vi "closeMethodViReference.vi"(8 "error in (no error)":errorcluster, 11 "TestCase in":refnum<class "TestCase.lvclass">) -> (0 "error out":errorcluster, 3 "TestCase in":refnum<class "TestCase.lvclass">)   [LabVIEW 2011, in "TestCase.lvclass"]
uses:
  TestCase.lvclass
  TestCase.lvclass/TestCase.ctl
panel:
  # "JKI VI Tester for LabVIEW\nhttp://jkisoft.com/vi-tester\nCopyright (C) 2007-2009, JKI <info@jkisoft.com>\nALL RIGHTS RESERVED"
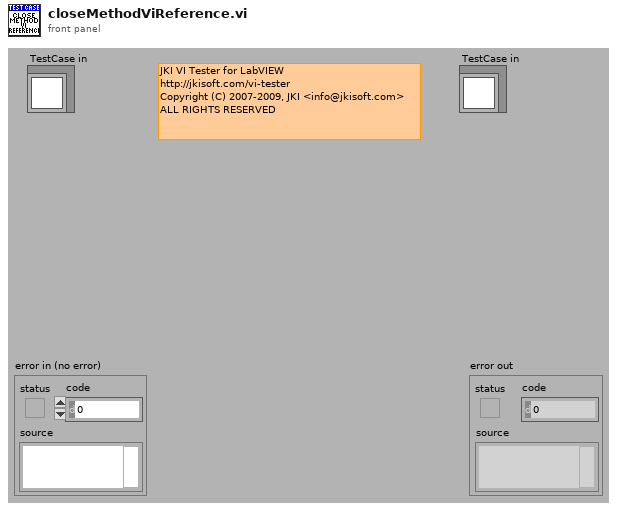
[diagram p1: front panel]
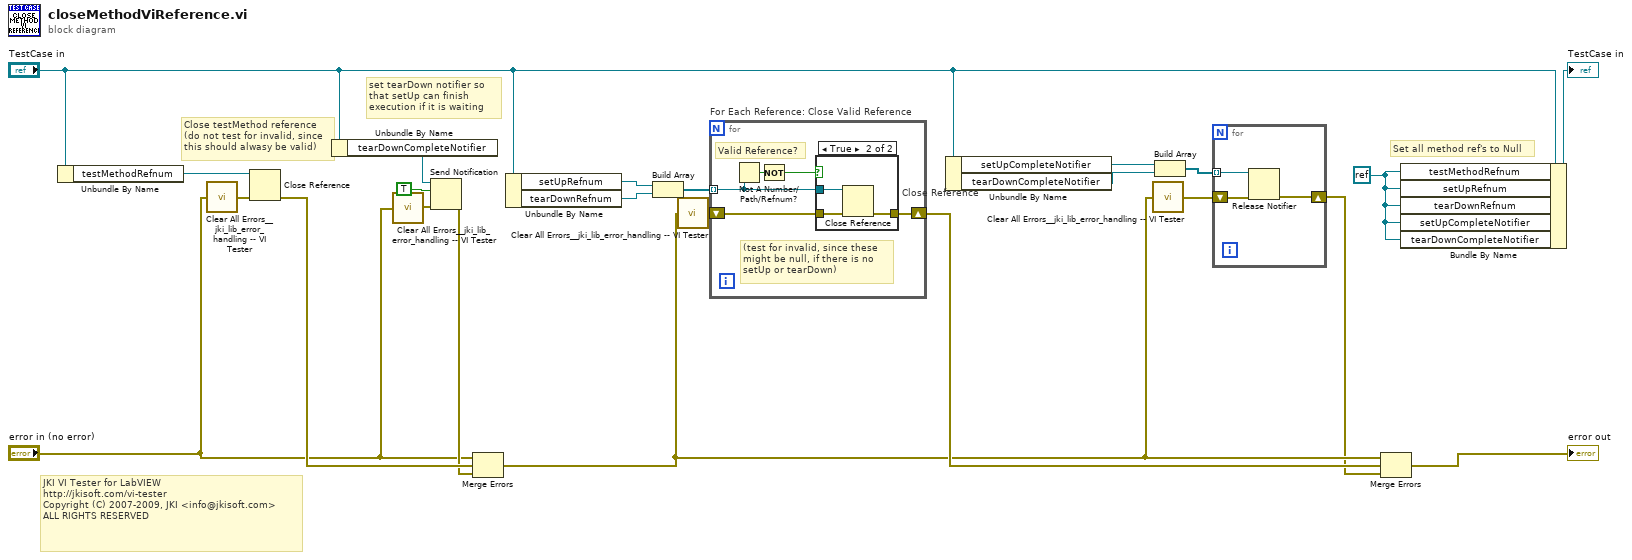
[diagram p0: block diagram]
diagram:
  w7 = refnum<k0> refnum
  # "JKI VI Tester for LabVIEW\nhttp://jkisoft.com/vi-tester\nCopyright (C) 2007-2009, JKI <info@jkisoft.com>\nALL RIGHTS RESERVED"
  # "set tearDown notifier so that setUp can finish execution if it is waiting"
  # "Close testMethod reference\n(do not test for invalid, since this should alwasy be valid)"
  # "Set all method ref's to Null"
  n1 = Unbundle By Name("TestCase in") -> ("testMethodRefnum"=w22:refnum<vi>)
  n2 = call "Clear All Errors__jki_lib_error_handling -- VI Tester.vi"("error in"="error in (no error)") -> ("no error out"=w21:errorcluster)  [unwired: 4 in]
  n3 = Close Reference(reference=w22, error in (no error)=w21) -> (error out=w20:errorcluster)
  n4 = Unbundle By Name("TestCase in") -> ("tearDownCompleteNotifier"=w4:refnum<notifier>)
  n5 = call "Clear All Errors__jki_lib_error_handling -- VI Tester.vi"("error in"="error in (no error)") -> ("no error out"=w2:errorcluster)  [unwired: 4 in]
  n6 = Send Notification(notification=TRUE, notifier=w4, error in (no error)=w2) -> (error out=w3:errorcluster)  [unwired: 1 out]
  n7 = Merge Errors("error in (no error)", w20, w3) -> (w10:errorcluster)
  n8 = Unbundle By Name("TestCase in") -> ("setUpRefnum"=w19:refnum<vi>, "tearDownRefnum"=w18:refnum<vi>)
  n9 = Build Array(w19, w18) -> (w16:refnum<vi>[])
  n10 = call "Clear All Errors__jki_lib_error_handling -- VI Tester.vi"("error in"=w10) -> ("no error out"=w17:errorcluster)  [unwired: 4 in]
  n11 = for "For Each Reference: Close Valid Reference" {
    shift-right: [w27] -> w15
    shift-left: w17 -> [w28]
    tunnel: w16 -> [w25] mode=indexing
    # "(test for invalid, since these might be null, if there is no setUp or tearDown)"
    # "Valid Reference?"
    n12 = Not A Number/Path/Refnum?(number/path/refnum=w25) -> (NaN/Path/Refnum?=w26:bool)
    n13 = Not(x=w26) -> (.not. x?=w24:bool)
    n14 = case "Close Reference" shown="True" w24 {
      tunnel: w28 -> [w29 w32]
      tunnel: w25 -> [_ w31]
      tunnel: [w29 w30] -> w27
      frame False {
      }
      frame True {
        n15 = Close Reference(reference=w31, error in (no error)=w32) -> (error out=w30:errorcluster)
      }
    }
  }
  n16 = Unbundle By Name("TestCase in") -> ("setUpCompleteNotifier"=w13:refnum<notifier>, "tearDownCompleteNotifier"=w12:refnum<notifier>)
  n17 = call "Clear All Errors__jki_lib_error_handling -- VI Tester.vi"("error in"=w10) -> ("no error out"=w9:errorcluster)  [unwired: 4 in]
  n18 = Build Array(w13, w12) -> (w11:refnum<notifier>[])
  n19 = for {
    tunnel: w11 -> [w35] mode=indexing
    shift-right: [w34] -> w8
    shift-left: w9 -> [w33]
    n20 = Release Notifier(notifier=w35, error in (no error)=w33) -> (error out=w34:errorcluster)  [unwired: 1 in, 2 out]
  }
  n21 = Merge Errors(w10, w15, w8) -> (→"error out":errorcluster)
  n22 = Bundle By Name(cluster="TestCase in", "testMethodRefnum"=w7, "setUpRefnum"=w7, "tearDownRefnum"=w7, "setUpCompleteNotifier"=w7, "tearDownCompleteNotifier"=w7) -> (→"TestCase in":refnum<class "TestCase.lvclass">)
